vi "4Pi Dual DM - 1D Gaussian.vi"(0 "Parameters In":dbl[](array[numeric]), 2 "Number of Points":dbl=1000.0 format="%#_13g", 9 "Max X Value":dbl, 11 "Min X Value":dbl) -> (6 "X Values":dbl[](array[numeric]), 10 "Y Values":dbl[](array[numeric]))   [LabVIEW 2021]
doc: "Baed on the input parameters this function generates a 1D Gaussian following the same formula as LabVIEW uses for the Gaussian Fitting VI. The Output is a 1D array of X values and a 1D array of Y values. \n\nThe Parameters In array assumes the following order:\n\nAmplitude\nCenter Position\nSigma (Width)\nOffset"
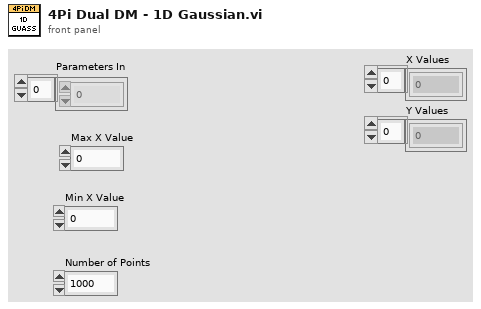
[diagram p1: front panel]
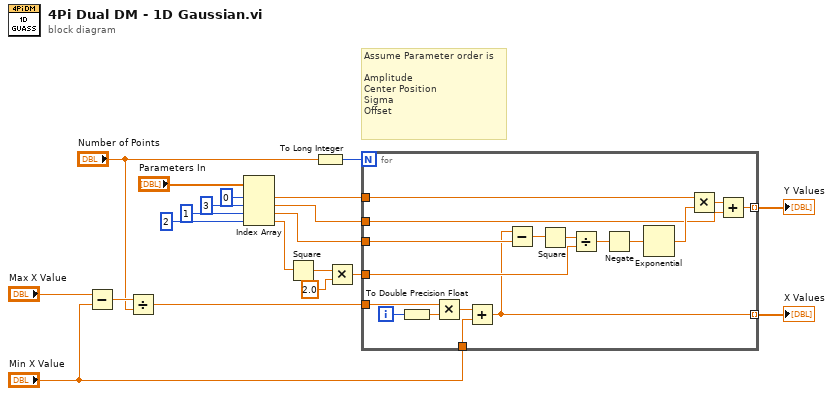
[diagram p0: block diagram]
diagram:
  # "Assume Parameter order is\n\nAmplitude\nCenter Position\nSigma\nOffset"
  n1 = Subtract(x="Max X Value", y="Min X Value") -> (x-y=w17:dbl)
  n2 = Divide(x=w17, y="Number of Points") -> (x/y=w16:dbl)
  n3 = Index Array(array="Parameters In", index #1=0 ("index"), index #2=3 ("index"), index #3=1 ("index"), index #4=2 ("index")) -> (element #1=w4:dbl, element #2=w3:dbl, element #3=w2:dbl, element #4=w1:dbl)
  n4 = Square(x=w1) -> (x^2=w20:dbl)
  n5 = To Long Integer(number="Number of Points") -> (32bit integer=w14:i32)
  n6 = Multiply(x=w20, y=2.0) -> (x*y=w18:dbl)
  n7 = for {
    N: w14 -> [_]
    tunnel: w4 -> [w37]
    tunnel: w2 -> [w36]
    tunnel: w3 -> [w29]
    tunnel: w18 -> [w33]
    tunnel: [w28] -> w10 mode=indexing
    tunnel: w16 -> [w25]
    tunnel: "Min X Value" -> [w23]
    tunnel: [w22] -> w11 mode=indexing
    i -> [w27]
    n8 = To Double Precision Float(number=w27) -> (double precision float=w26:dbl)
    n9 = Multiply(x=w25, y=w26) -> (x*y=w24:dbl)
    n10 = Add(x=w24, y=w23) -> (x+y=w22:dbl)
    n11 = Subtract(x=w22, y=w36) -> (x-y=w35:dbl)
    n12 = Square(x=w35) -> (x^2=w34:dbl)
    n13 = Divide(x=w34, y=w33) -> (x/y=w21:dbl)
    n14 = Negate(x=w21) -> (-x=w32:dbl)
    n15 = Exponential(1:w32) -> (0:w31:dbl)
    n16 = Multiply(x=w37, y=w31) -> (x*y=w30:dbl)
    n17 = Add(x=w30, y=w29) -> (x+y=w28:dbl)
  }
  "X Values" <- w11
  "Y Values" <- w10
